vi "Log.vi"(8 "error in (no error)":errorcluster, 9 "Timestamp data points":bool, 10 "tdms file":refnum<k34>, 11 "Combined Result in":refnum<class "Combined Result.lvclass">) -> (0 "error out":errorcluster, 2 "tdms file out":refnum<k34>, 3 "Combined Result out":refnum<class "Combined Result.lvclass">)   [LabVIEW 2021, in "Combined Result.lvclass"]
uses:
  Combined Result.lvclass
  Combined Result.lvclass/Combined Result.ctl
  Acquired Result/Acquired Result.lvclass
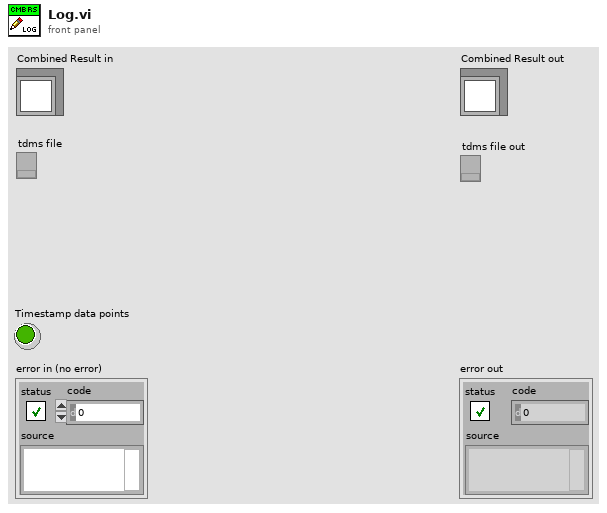
[diagram p1: front panel]
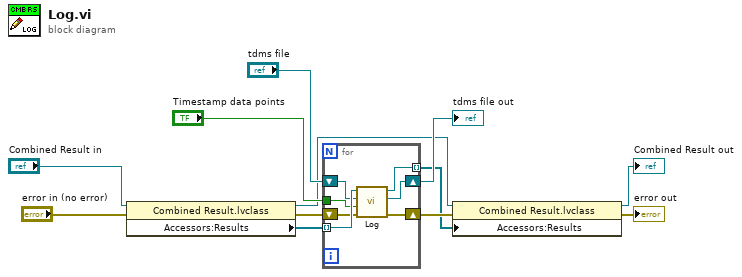
[diagram p0: block diagram]
diagram:
  n1 = property class="Combined Result.lvclass"(reference="Combined Result in", error in="error in (no error)") -> (reference out=w2:refnum<class "Combined Result.lvclass">, error out=w7:errorcluster, "Accessors:Results"=w3:refnum<class "Acquired Result.lvclass">[])
  n2 = for {
    tunnel: "Timestamp data points" -> [w13]
    tunnel: w3 -> [w17] mode=indexing
    tunnel: [w18] -> w1 mode=indexing
    shift-right: [w14] -> w11
    shift-left: "tdms file" -> [w15]
    shift-right: [w19] -> w12
    shift-left: w7 -> [w16]
    n3 = call-dynamic "Log.vi"("error in (no error)"=w16, "Timestamp data points"=w13, "tdms file"=w15, "Acquired Result in"=w17) -> ("error out"=w19:errorcluster, "tdms file out"=w14:refnum<k34>, "Acquired Result out"=w18:refnum<class "Acquired Result.lvclass">)  [unwired: 5 in]
  }
  "tdms file out" <- w11
  n4 = property class="Combined Result.lvclass"(reference=w2, error in=w12, "Accessors:Results"=w1) -> (reference out=→"Combined Result out":refnum<class "Combined Result.lvclass">, error out=→"error out":errorcluster)
